vi "Local Buffer Loop Async.vi"(10 "ExecAnchor":refnum<class "ExecAnchor.lvclass">, 11 "LocalGraphBuffer in":refnum<class "LocalGraphBuffer.lvclass">) -> ()   [LabVIEW 2020, in "VolatusGUIElements.lvlib" / "LocalGraphBuffer.lvclass"]
uses:
  LocalGraphBuffer.lvclass
  lv-exec-anchor/ExecAnchor/ExecAnchor.lvclass
  LocalGraphBuffer.lvclass/LocalGraphBuffer.ctl
  lv-exec-anchor/ExecAnchor/ExecAnchor.lvclass/ExecAnchor.ctl
  lv-vecto/Vecto/Channel DBL/Channel DBL.lvclass/Channel DBL.ctl
  lv-vecto/Vecto/Group DBL/Value by Index.vi
  lv-vecto/Vecto/Channel DBL/Channel DBL.lvclass
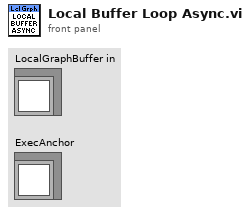
[diagram p1: front panel]
types:
  T1 = typedef "VolatusGUIElements.lvlib/LocalGraphBuffer.lvclass/Plot.ctl" = cluster{"Data Q":refnum<queue>, "Time Q":refnum<queue>, "Group":string, "Channel Index":i32, "Local":bool, "Channel":refnum<class "Channel DBL.lvclass">}
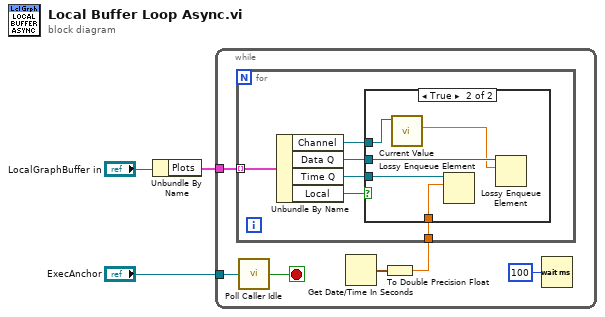
[diagram p0: block diagram]
diagram:
  n1 = Unbundle By Name("LocalGraphBuffer in") -> ("Plots"=w2:T1[])
  n2 = while {
    tunnel: w2 -> [w8]
    tunnel: "ExecAnchor" -> [w7]
    stop <- w6 stop-if-true
    n3 = call "Poll Caller Idle.vi"("ExecAnchor in"=w7) -> ("Caller Idle"=w6:bool)  [unwired: 3 in, 1 out]
    n4 = Get Date/Time In Seconds() -> (seconds since 1Jan1904=w5:timestamp)
    n5 = To Double Precision Float(number=w5) -> (double precision float=w4:dbl)
    n6 = for {
      tunnel: w8 -> [w15] mode=indexing
      tunnel: w4 -> [w10]
      n7 = Unbundle By Name(w15) -> ("Channel"=w11:refnum<class "Channel DBL.lvclass">, "Data Q"=w12:refnum<queue>, "Time Q"=w13:refnum<queue>, "Local"=w14:bool)
      n8 = case shown="True" w14 {
        tunnel: w13 -> [_ w20]
        tunnel: w12 -> [_ w18]
        tunnel: w11 -> [_ w19]
        tunnel: w10 -> [_ w16]
        frame False {
        }
        frame True {
          n9 = call "Current Value.vi"("Channel in"=w19) -> ("Scaled"=w17:dbl)  [unwired: 6 in, 4 out]
          n10 = Lossy Enqueue Element(queue=w20, element=w16) -> ()  [unwired: 1 in, 4 out]
          n11 = Lossy Enqueue Element(queue=w18, element=w17) -> ()  [unwired: 1 in, 4 out]
        }
      }
    }
    n12 = Wait (ms)(milliseconds to wait=u32 100) -> ()  [unwired: 1 out]
  }
